vi "Check existence.vi"(0 "Data.PG":refnum<class "LV-Data.PGSQL.lvclass">=refnum, 1 "Table path":string, 2 "column name":string, 3 "error in (no error)":errorcluster, 4 "Numeric":i32) -> (5 "Data.PG out":refnum<class "LV-Data.PGSQL.lvclass">, 6 "Boolean":bool, 7 "error out":errorcluster)   [LabVIEW 2016, in "LV-Data.PGSQL.lvclass"]
uses:
  LV-Data.PGSQL.lvclass
  <vilib>/JDP Science/PostgreSQL Library/Connection/PQ Connection.lvclass
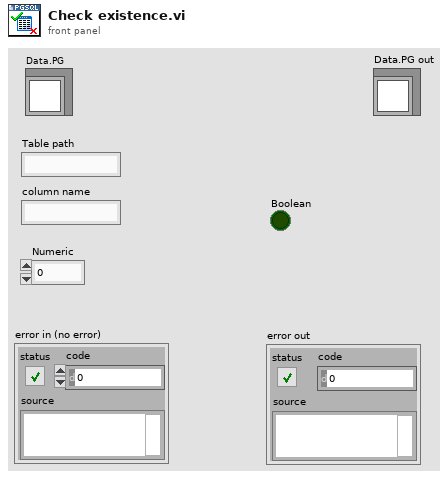
[diagram p1: front panel]
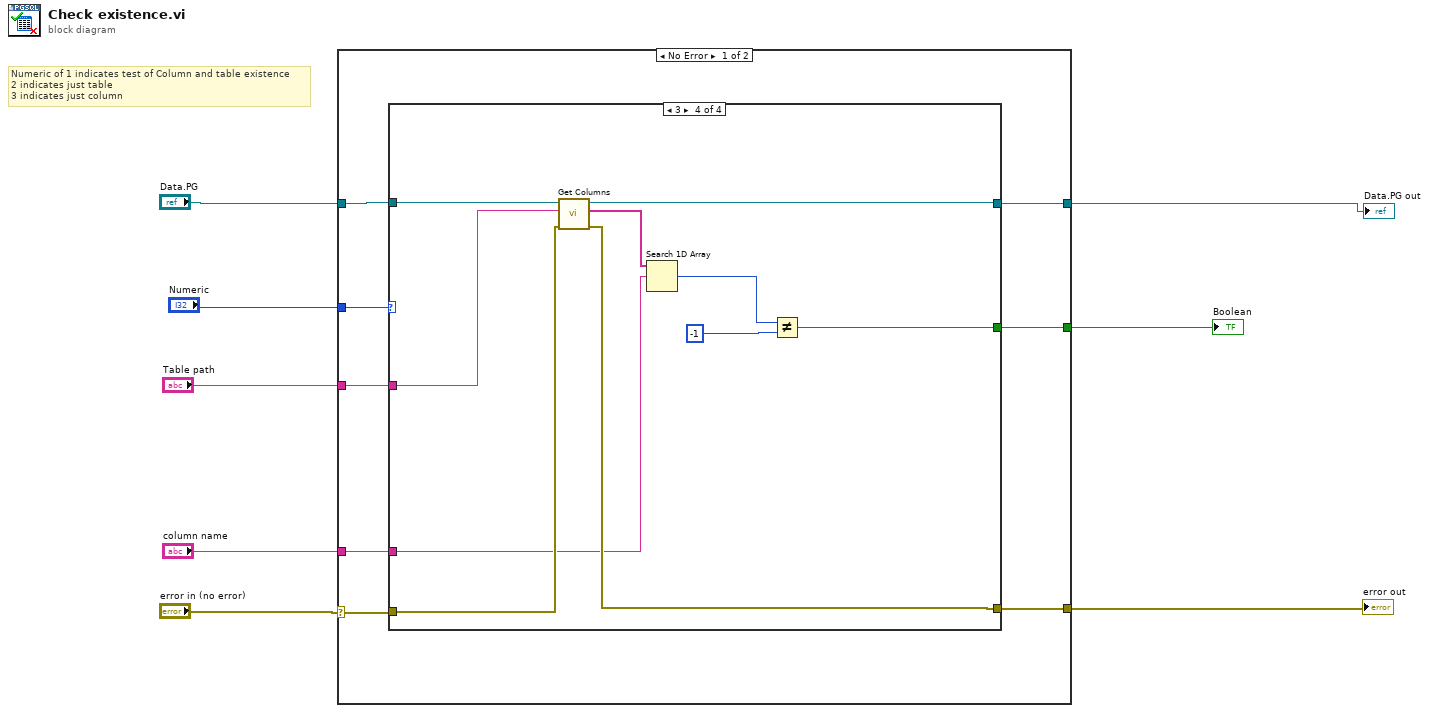
[diagram p0: block diagram]
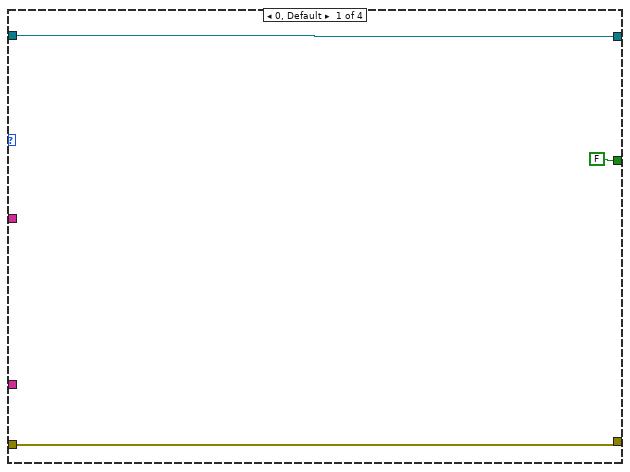
[diagram p2: hidden frame]
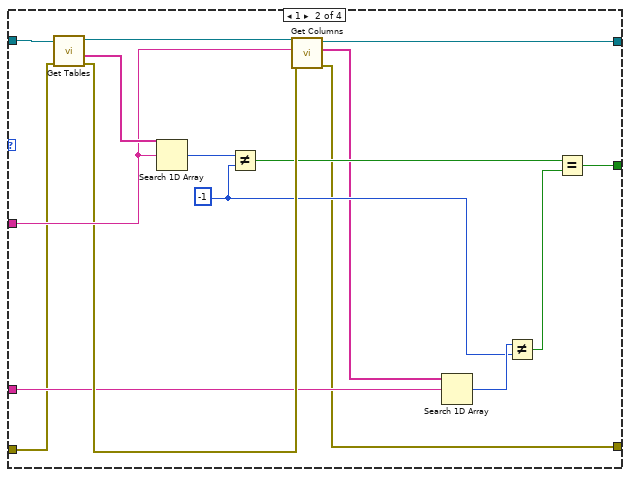
[diagram p3: hidden frame]
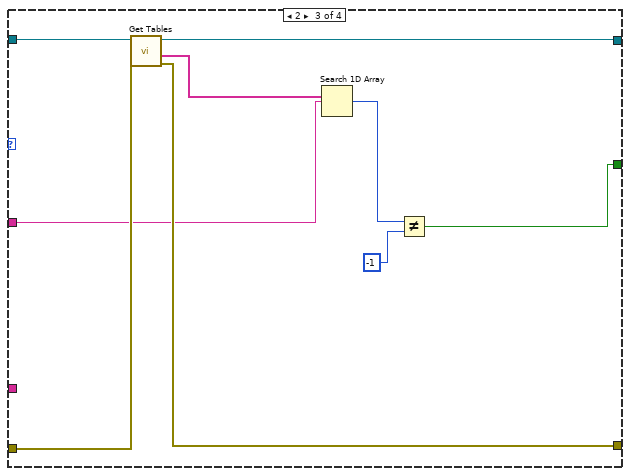
[diagram p4: hidden frame]
diagram:
  # "Numeric of 1 indicates test of Column and table existence \n2 indicates just table \n3 indicates just column"
  n1 = case shown="No Error" "error in (no error)" {
    selector: "error in (no error)" -> [w9 w56]
    tunnel: "Numeric" -> [w16 _]
    tunnel: "Data.PG" -> [w15 w55]
    tunnel: "Table path" -> [w14 _]
    tunnel: [w13 _] -> w5
    tunnel: [w12 w55] -> w4
    tunnel: [w11 w56] -> w3
    tunnel: "column name" -> [w10 _]
    frame No Error {
      n2 = case shown="3" w16 {
        tunnel: w15 -> [w18 w35 w42 w53]
        tunnel: w9 -> [w17 w21 w40 w51]
        tunnel: w14 -> [_ w32 w37 w46]
        tunnel: [FALSE w24 w36 w48] -> w13
        tunnel: [w18 w22 w41 w52] -> w12
        tunnel: [w17 w23 w39 w50] -> w11
        tunnel: w10 -> [_ w29 _ w47]
        frame 0, Default {
        }
        frame 1 {
          w27 = -1 ("y")
          n3 = call "Get Tables.vi"("error in (no error)"=w21, "Data.PG"=w35) -> ("error out"=w30:errorcluster, "Table Paths"=w34:string[], "Data.PG out"=w31:refnum<class "LV-Data.PGSQL.lvclass">)  [unwired: 6 in, 1 out]
          n4 = Search 1D Array(1D array=w34, element=w32) -> (index of element=w33:i32)  [unwired: 1 in]
          n5 = Not Equal?(x=w33, y=w27) -> (x != y?=w25:bool)
          n6 = call "Get Columns.vi"("error in (no error)"=w30, "selected table path"=w32, "Data.PG in"=w31) -> ("error out"=w23:errorcluster, "Column Names"=w20:string[], "Data.PG out"=w22:refnum<class "LV-Data.PGSQL.lvclass">)  [unwired: 4 in, 2 out]
          n7 = Search 1D Array(1D array=w20, element=w29) -> (index of element=w28:i32)  [unwired: 1 in]
          n8 = Not Equal?(x=w28, y=w27) -> (x != y?=w26:bool)
          n9 = Equal?(x=w25, y=w26) -> (x = y?=w24:bool)
        }
        frame 2 {
          n10 = call "Get Tables.vi"("error in (no error)"=w40, "Data.PG"=w42) -> ("error out"=w39:errorcluster, "Table Paths"=w43:string[], "Data.PG out"=w41:refnum<class "LV-Data.PGSQL.lvclass">)  [unwired: 6 in, 1 out]
          n11 = Search 1D Array(1D array=w43, element=w37) -> (index of element=w44:i32)  [unwired: 1 in]
          n12 = Not Equal?(x=w44, y=-1) -> (x != y?=w36:bool)
        }
        frame 3 {
          n13 = call "Get Columns.vi"("error in (no error)"=w51, "selected table path"=w46, "Data.PG in"=w53) -> ("error out"=w50:errorcluster, "Column Names"=w45:string[], "Data.PG out"=w52:refnum<class "LV-Data.PGSQL.lvclass">)  [unwired: 4 in, 2 out]
          n14 = Search 1D Array(1D array=w45, element=w47) -> (index of element=w54:i32)  [unwired: 1 in]
          n15 = Not Equal?(x=w54, y=-1) -> (x != y?=w48:bool)
        }
      }
    }
    frame Error {
    }
  }
  "Boolean" <- w5
  "Data.PG out" <- w4
  "error out" <- w3
